vi "To Cleanup Initialize and Close Session Behavior.vi"(11 "initialize and close session behavior":T1) -> (3 "cleanup initialize and close session behavior":T1)   [LabVIEW 2020, in "MeasurementLink Instrument.lvlib" / "IInstrument.lvclass"]
uses:
  Initialize and Close Session Behavior.ctl
  IInstrument.lvclass
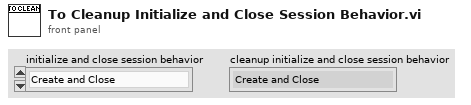
[diagram p1: front panel]
types:
  T1 = typedef "MeasurementLink Instrument.lvlib/IInstrument.lvclass/Initialize and Close Session Behavior.ctl" = enum16{"Create and Close", "Attach and Detach", "Create and Detach", "Attach and Close"}
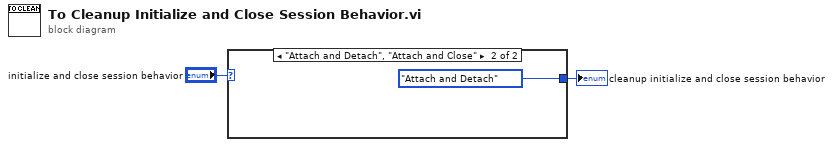
[diagram p0: block diagram]
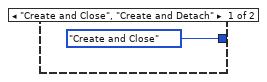
[diagram p2: hidden frame]
diagram:
  n1 = case shown="\"Attach and Detach\", \"Attach and Close\"" "initialize and close session behavior" {
    tunnel: [Initialize_and_Close_Session_Behavior."Create and Close" ("cleanup initialize and close session behavior") Initialize_and_Close_Session_Behavior."Attach and Detach" ("cleanup initialize and close session behavior")] -> w1
    frame "Create and Close", "Create and Detach" {
    }
    frame "Attach and Detach", "Attach and Close" {
    }
  }
  "cleanup initialize and close session behavior" <- w1
